vi "Test Zentral Trigger PC nur Mira Sync.vi"() -> ()   [LabVIEW 2009, in "POLARIS BME DG.lvlib"]
uses:
  POLARIS BME DG.lvlib
  LV-BME Interface/ChnlSettings.ctl
  LV-BME Interface/BME_DG_TriggerSettings.ctl
  DG Classes/BME_DG_G05P2/SG05P2 Clock and Trigger Settings.ctl
  LV-BME Interface/ClockSource.ctl
  DG Classes/BME_DG_G05P2/BME_DG_G05P2.lvclass
  DG Classes/BME_DG_G05P2_Chnl/BME_DG_G05P2_Chnl.lvclass
  ChnlParam.ctl
  DG Classes/BME_DG_System/BME_DG_System.lvclass
  DG Classes/BME_DG_Base/BME_DG_Base.lvclass
  DG Classes/BME_DG_Chnl/BME_DG_Chnl.lvclass
panel:
  in  "pathParameterFile":path=path "C:/CS Framework/LVSCC/LV2009/GPL/Projects/cs-framework/CSClass/CSPOLARIS/POLARIS BME DG/tset config  file.xml"
  out "stop error":errorcluster
  in  "Karten Parameter":T1[](array[typedef])=[{"Trigger"={"InputTerminated?"=TRUE, "InternalClockPeriode(µs)"=100000.0, "TriggerLevel"=1.8999000000000001, "PresetValue"=0, "DivideBy"=0, "Clock Source"=1, "Gate Divider"=1, "PositiveGate?"=TRUE, "InternalTrigger?"=TRUE, "InternalArm?"=FALSE, "SWTrigger?"=FALSE, "RisingEdge?"=FALSE, "StopOnPreset?"=FALSE, "ResetWhenDone?"=TRUE, "TriggerEnabled?"=TRUE}, "ClockSource "=1, "V2 Trigger Settings"={"Gate Type"=TRUE, "Synchronize Gate"=FALSE, "Force Trigger (µs)"=0.0, "MS Bus"=1024}, " prescaller crst oscill."=8, "CardName"="Mira Sync"}] {"V2 Trigger Settings"."MS Bus" format="%04x" items=["Local Primary"=1, "Local Secondary"=2, "Local Force"=4, "Resynchronize"=8, "Master Primary"=16, "Master Secondary"=32, "Master Force"=64, "System Clock"=128, "Delay Clock"=256, "Inhibit Local"=512, "Start Local"=1024, "Start Bus"=2048, "Step Back Local"=4096, "Step Back Bus"=8192, "Enable From E"=65536, "Enable From F"=131072, "Enable From Bus"=262144]; "V2 Trigger Settings"."Force Trigger (µs)" min=0.0 format="%.6f"; "ClockSource" items=["Internal Oscillator"=1, "External Trigger"=2, "Trigger & Oscillator"=3, "MasterSlave Bus"=4]; "Trigger"."Gate Divider" min=1 max=1000000; "Trigger"."Clock Source" items=["Internal Oscillator"=1, "External Trigger"=2, "Trigger & Oscillator"=3]; "Trigger"."InternalClockPeriode(µs)" format="%#_11g"}
  in  "Go Signal":u32(ring)=1 items=["Local Primary"=1, "Local Secondary"=2, "Local Force"=4, "Resynchronize"=8, "Master Primary"=16, "Master Secondary"=32, "Master Force"=64, "System Clock"=128, "Delay Clock"=256, "Inhibit Local"=512, "Start Local"=1024, "Start Bus"=2048, "Step Back Local"=4096, "Step Back Bus"=8192, "From E"=65536, "From F"=131072, "From Bus"=262144]
  out "Problem Chnls out":string[](array[string])
  out "DelayFormulas":string[](array[string])=["0.0", "", ""]
  in  "Reset Error":bool
  out "error out":errorcluster
  in  "Update Delay formula":bool=TRUE
  in  "DelayFormula":string="0.0"
  in  "Aknowledge interrupts":bool=TRUE
  in  "stop 3":bool=TRUE
  in  "SetDelay":bool=TRUE
  in  "UpdateChnl":bool=TRUE
  in  "ChnlParameter":T5 {"ChnParam2write"."Delay (µs)" min=0.0 max=100000000.0 format="%.5f"}
  out "CountsRemains":i32=2147483647
  out "TriggerCounters":i32[](array[numeric])=[0, 0, 0, 0, 0, -533591008, 0, 0, 0, 0]
  out "Interrupts":u32[](array[numeric])=[11008, 11008, 10240, 11008, 11008, 11008, 11008, 10240, 10240, 10240] format="%b"
  out "RemainingTriggers":T6(array[cluster])=[[{"Time Stamp"=timestamp(3421635734.171875 s since 1904-01-01), "Numeric"=1}, {"Time Stamp"=timestamp(3421635734.171875 s since 1904-01-01), "Numeric"=1}, {"Time Stamp"=timestamp(3421635734.171875 s since 1904-01-01), "Numeric"=1}, {"Time Stamp"=timestamp(3421635734.171875 s since 1904-01-01), "Numeric"=1}, {"Time Stamp"=timestamp(3421635734.171875 s since 1904-01-01), "Numeric"=1}, {"Time Stamp"=timestamp(3421635734.171875 s since 1904-01-01), "Numeric"=1}, {"Time Stamp"=timestamp(3421635734.171875 s since 1904-01-01), "Numeric"=1}, {"Time Stamp"=timestamp(3421635734.171875 s since 1904-01-01), "Numeric"=1}, {"Time Stamp"=timestamp(3421635734.171875 s since 1904-01-01), "Numeric"=1}, {"Time Stamp"=timestamp(3421635734.171875 s since 1904-01-01), "Numeric"=1}], [{"Time Stamp"=timestamp(3421635734.171875 s since 1904-01-01), "Numeric"=1}, {"Time Stamp"=timestamp(3421635734.171875 s since 1904-01-01), "Numeric"=1}, {"Time Stamp"=timestamp(3421635734.171875 s since 1904-01-01), "Numeric"=1}, {"Time Stamp"=timestamp(3421635734.171875 s since 1904-01-01), "Numeric"=1}, {"Time Stamp"=timestamp(3421635734.171875 s since 1904-01-01), "Numeric"=1}, {"Time Stamp"=timestamp(3421635734.171875 s since 1904-01-01), "Numeric"=1}, {"Time Stamp"=timestamp(3421635734.171875 s since 1904-01-01), "Numeric"=1}, {"Time Stamp"=timestamp(3421635734.171875 s since 1904-01-01), "Numeric"=1}, {"Time Stamp"=timestamp(3421635734.171875 s since 1904-01-01), "Numeric"=1}, {"Time Stamp"=timestamp(3421635734.171875 s since 1904-01-01), "Numeric"=1}], [{"Time Stamp"=timestamp(3421635734.171875 s since 1904-01-01), "Numeric"=1}, {"Time Stamp"=timestamp(3421635734.171875 s since 1904-01-01), "Numeric"=1}, {"Time Stamp"=timestamp(3421635734.171875 s since 1904-01-01), "Numeric"=1}, {"Time Stamp"=timestamp(3421635734.171875 s since 1904-01-01), "Numeric"=1}, {"Time Stamp"=timestamp(3421635734.171875 s since 1904-01-01), "Numeric"=1}, {"Time Stamp"=timestamp(3421635734.171875 s since 1904-01-01), "Numeric"=1}, {"Time Stamp"=timestamp(3421635734.171875 s since 1904-01-01), "Numeric"=1}, {"Time Stamp"=timestamp(3421635734.171875 s since 1904-01-01), "Numeric"=1}, {"Time Stamp"=timestamp(3421635734.171875 s since 1904-01-01), "Numeric"=1}, {"Time Stamp"=timestamp(3421635734.171875 s since 1904-01-01), "Numeric"=1}]] {"Time Stamp" format="%<%I:%M:%S%3u %p>T"}
  in  "stop 2":bool=TRUE
  in  "ReadStatus":bool=TRUE
  in  "Activate":bool=TRUE
  in  "ResetModuloCounters":bool=TRUE
  in  "TriggerModulo":u32=4
  out "Modulo Settings":u32[](array[numeric])=[1, 1, 1]
  out "Chnls":T4[](array[typedef])=[{" Delay (µs)"=0.0, "On? (false)"=TRUE, "PositiveVoltage?"=TRUE, "50OhmTerminated? "=TRUE, "25OhmOutput?"=FALSE}, {" Delay (µs)"=0.0, "On? (false)"=TRUE, "PositiveVoltage?"=TRUE, "50OhmTerminated? "=TRUE, "25OhmOutput?"=FALSE}, {" Delay (µs)"=0.0, "On? (false)"=TRUE, "PositiveVoltage?"=TRUE, "50OhmTerminated? "=TRUE, "25OhmOutput?"=FALSE}] {"Delay (µs)" min=0.0 max=100000000.0 format="%.5f"}
  in  "Trigger Base":T2={"InputTerminated?"=TRUE, "InternalClockPeriode(µs)"=100000.0, "TriggerLevel"=-0.1001, "PresetValue"=0, "DivideBy"=4, "Clock Source"=1, "Gate Divider"=1, "PositiveGate?"=TRUE, "InternalTrigger?"=TRUE, "InternalArm?"=FALSE, "SWTrigger?"=FALSE, "RisingEdge?"=FALSE, "StopOnPreset?"=FALSE, "ResetWhenDone?"=TRUE, "TriggerEnabled?"=TRUE} {"Gate Divider" min=1 max=1000000; "Clock Source" items=["Internal Oscillator"=1, "External Trigger"=2, "Trigger & Oscillator"=3]; "InternalClockPeriode(µs)" format="%#_11g"}
  in  "Selected Chnl":u16(ring) items=["18 MHz", "A", "B"]
  in  "Selected Card":u16(ring) items=["Mira Sync"]
  in  "STOP":bool=TRUE
  in  "ChnParam2write":T4={" Delay (µs)"=0.0, "On? (false)"=TRUE, "PositiveVoltage?"=TRUE, "50OhmTerminated? "=TRUE, "25OhmOutput?"=FALSE} {"Delay (µs)" min=0.0 max=100000000.0 format="%.5f"}
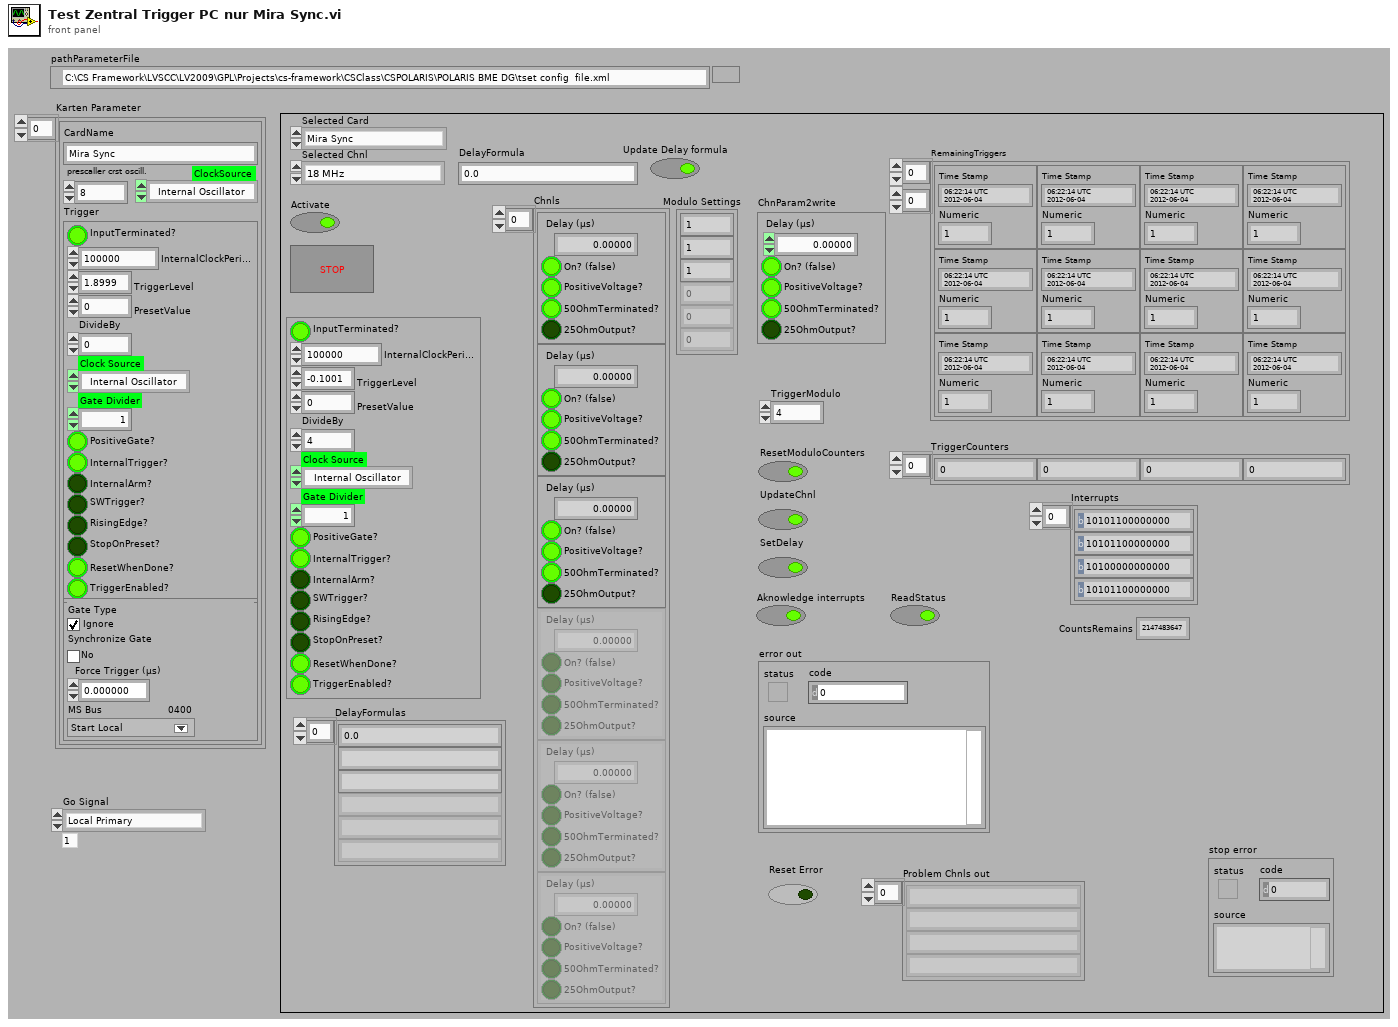
[diagram p1: front panel]
types:
  T1 = typedef "SG05P2 Clock and Trigger Settings.ctl" = cluster{"Trigger":T2, "ClockSource ":T3, "V2 Trigger Settings":cluster{"Gate Type":bool, "Synchronize Gate":bool, "Force Trigger (µs)":dbl, "MS Bus":u32}, " prescaller crst oscill.":u32, "CardName":string}
  T2 = typedef "POLARIS BME DG.lvlib/BME_DG_TriggerSettings.ctl" = cluster{"InputTerminated?":bool, "InternalClockPeriode(µs)":dbl, "TriggerLevel":dbl, "PresetValue":i32, "DivideBy":i32, "Clock Source":u32, "Gate Divider":i32, "PositiveGate?":bool, "InternalTrigger?":bool, "InternalArm?":bool, "SWTrigger?":bool, "RisingEdge?":bool, "StopOnPreset?":bool, "ResetWhenDone?":bool, "TriggerEnabled?":bool}
  T3 = typedef "POLARIS BME DG.lvlib/ClockSource.ctl" = i32
  T4 = typedef "POLARIS BME DG.lvlib/ChnlSettings.ctl" = cluster{" Delay (µs)":dbl, "On? (false)":bool, "PositiveVoltage?":bool, "50OhmTerminated? ":bool, "25OhmOutput?":bool}
  T5 = cluster{"ChnlName":string, "ChnParam2write":T4, "TriggerModulo":u32}
  T6 = cluster{"Time Stamp":timestamp, "Numeric":i32}[][]
  T7 = typedef "ChnlParam.ctl" = cluster{"ChnlName":string, "DelayFormula":string, "OutputModulo":i32}
  T8 = cluster{"Gate Type":bool, "Synchronize Gate":bool, "Force Trigger (µs)":dbl, "MS Bus":u32}
  T9 = enum8{"Enabled", "Disabled", "Disabled and Grayed Out"}
  T10 = cluster{"ChnlName":string, "ChnParam2write":T4, "TriggerModulo":u32}[]
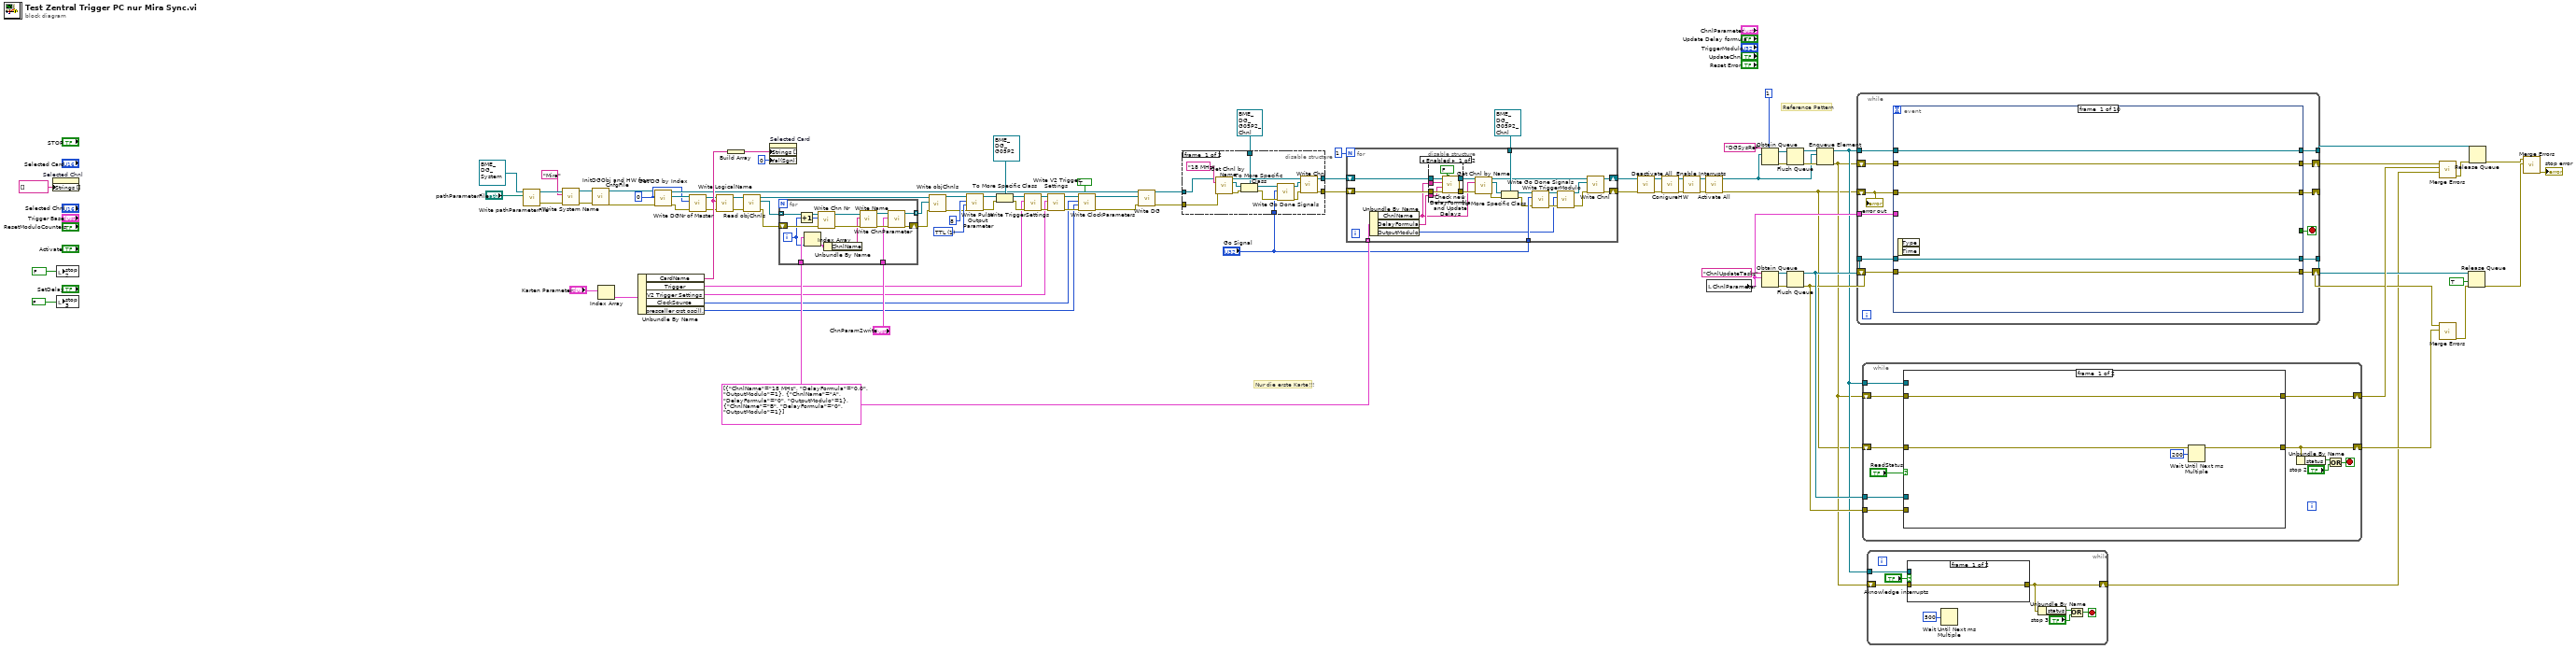
[diagram p0: block diagram]
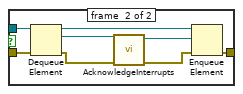
[diagram p4: hidden frame]
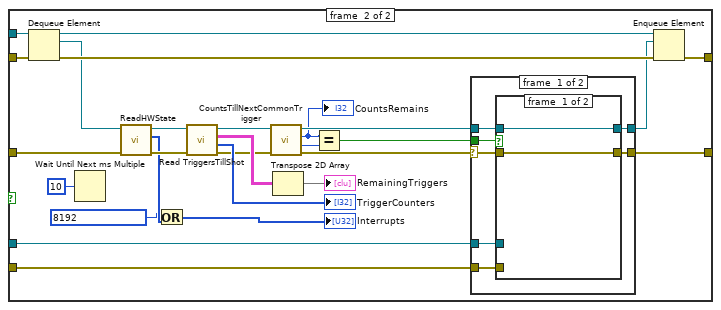
[diagram p5: hidden frame]
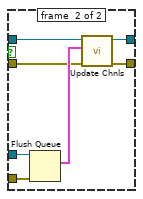
[diagram p6: hidden frame]
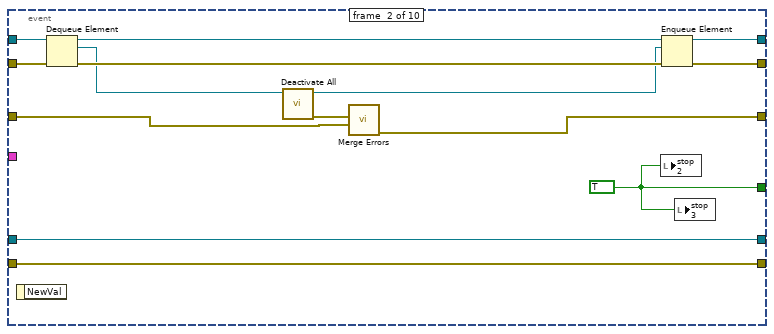
[diagram p8: hidden frame]
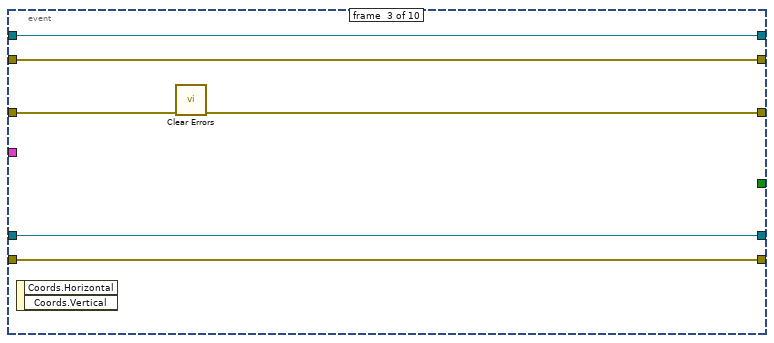
[diagram p9: hidden frame]
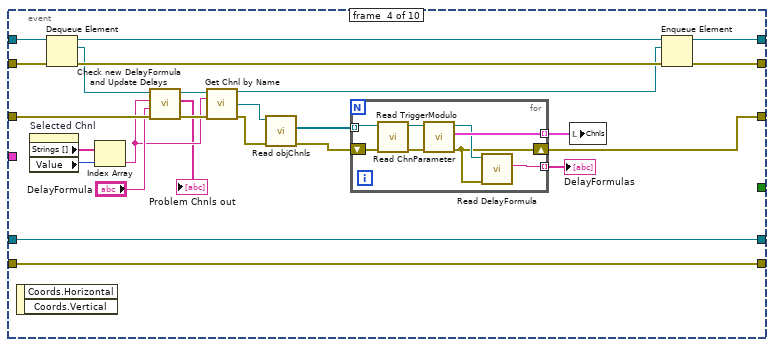
[diagram p10: hidden frame]
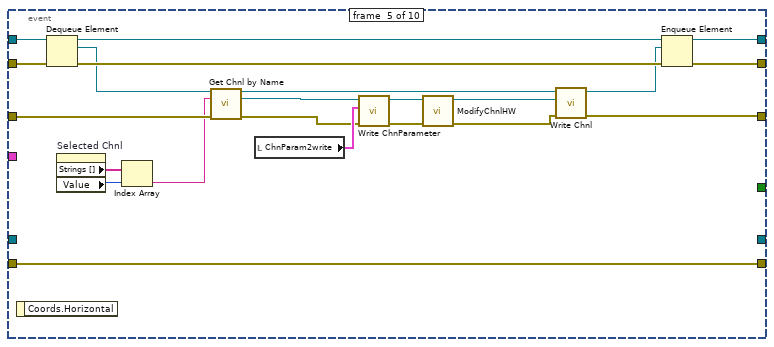
[diagram p11: hidden frame]
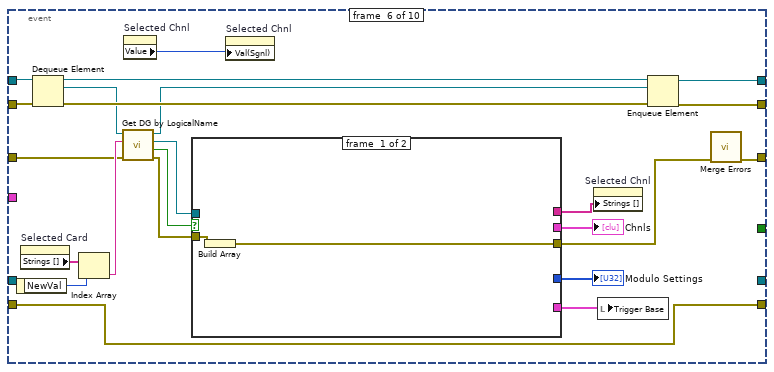
[diagram p12: hidden frame]
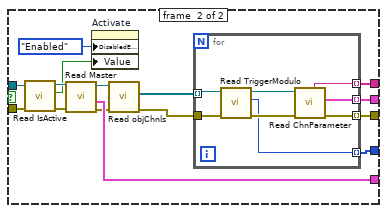
[diagram p13: hidden frame]
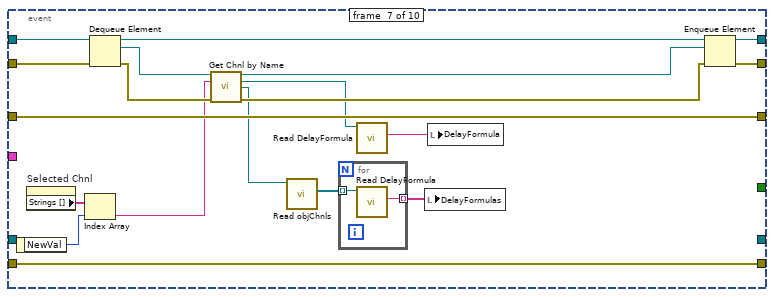
[diagram p14: hidden frame]
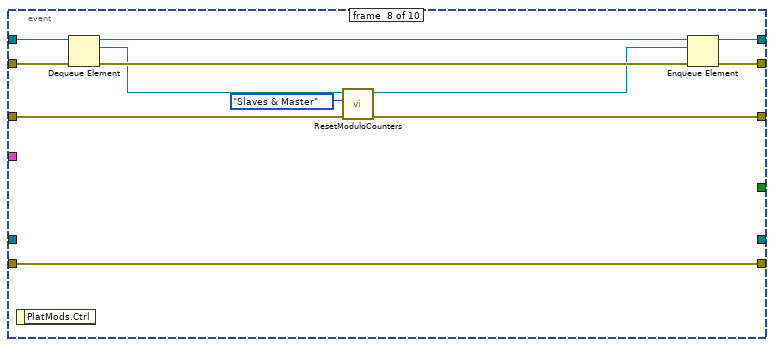
[diagram p15: hidden frame]
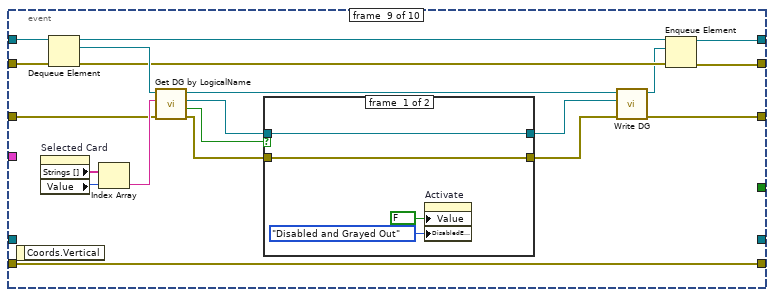
[diagram p16: hidden frame]
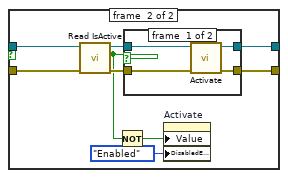
[diagram p17: hidden frame]
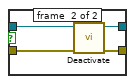
[diagram p18: hidden frame]
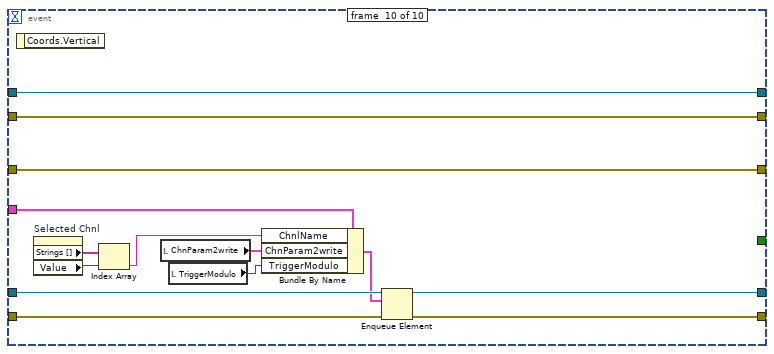
[diagram p19: hidden frame]
diagram:
  w31 = u32 1 items=["TTL"=1, "NIM"=2, "ECL"=3] ("Pulse Output Level")
  w46 = T7[] [{"ChnlName"="18 MHz", "DelayFormula"="0.0", "OutputModulo"=1}, {"ChnlName"="A", "DelayFormula"="0", "OutputModulo"=1}, {"ChnlName"="B", "DelayFormula"="0", "OutputModulo"=1}] ("ChnlParam 2")
  w10 = 0
  # "Nur die erste Karte!!!"
  # "Reference Pattern"
  n1 = property on="Selected Chnl" class="Ring (strict)"("Strings []"=string[] []) -> ()  [unwired: 2 in, 2 out]
  n2 = local write "stop 2"(FALSE ("stop 2")) -> ()
  n3 = local write "stop 3"(FALSE ("stop 3")) -> ()
  n4 = call-dynamic "Write pathParameterFile.vi"("pathParameterFile"="pathParameterFile", "BME_DG_System in"=refnum<class "BME_DG_System.lvclass"> refnum) -> ("error out"=w6:errorcluster, "BME_DG_System out"=w7:refnum<class "BME_DG_System.lvclass">)  [unwired: 8 in]
  n5 = call "Write System Name.vi"("error in (no error)"=w6, "log Name"="Mira", "BME_DG_System in"=w7) -> ("error out"=w3:errorcluster, "BME_DG_System out"=w4:refnum<class "BME_DG_System.lvclass">)  [unwired: 7 in]
  n6 = call "InitDGObj and HW from CnfgFile.vi"("error out"=w3, "BME_DG_System in"=w4) -> ("error IO"=w1:errorcluster, "BME_DG_System Out"=w2:refnum<class "BME_DG_System.lvclass">)  [unwired: 4 in]
  n7 = Index Array(array="Karten Parameter") -> (element=w14:T1)  [unwired: 1 in]
  n8 = Unbundle By Name(w14) -> ("CardName"=w72:string, "Trigger"=w18:T2, "V2 Trigger Settings"=w17:T8, "ClockSource"=w15:T3, "prescaller crst oscill."=w16:u32)
  n9 = call "Get DG by Index.vi"("error in (no error)"=w1, "index"=w10, "BME_DG_System in"=w2) -> ("error out"=w34:errorcluster, "BME_DG_Base.lvclass"=w37:refnum<class "BME_DG_Base.lvclass">, "BME_DG_System out"=w45:refnum<class "BME_DG_System.lvclass">)  [unwired: 6 in]
  n10 = call-dynamic "Write DGNr of Master.vi"("error in (no error)"=w34, "DGNr of Master"=w10, "BME_DG_Base in"=w37) -> ("error out"=w35:errorcluster, "BME_DG_Base out"=w36:refnum<class "BME_DG_Base.lvclass">)  [unwired: 7 in]
  n11 = call "Write LogicalName.vi"("error in (no error)"=w35, "LogicalName"=w72, "BME_DG_Base in"=w36) -> ("error out"=w38:errorcluster, "BME_DG_Base out"=w39:refnum<class "BME_DG_Base.lvclass">)  [unwired: 7 in]
  n12 = Build Array(w72) -> (w13:string[])
  n13 = call-dynamic "Read objChnls.vi"("error in (no error)"=w38, "BME_DG_Base in"=w39) -> ("error out"=w43:errorcluster, "objChnls"=w44:refnum<class "BME_DG_Chnl.lvclass">[], "BME_DG_Base out"=w41:refnum<class "BME_DG_Base.lvclass">)  [unwired: 6 in, 1 out]
  n14 = property on="Selected Card" class="Ring (strict)"("Strings []"=w13, "Val(Sgnl)"=u16 0 ("Value (Signaling)")) -> ()  [unwired: 2 in, 2 out]
  n15 = for {
    tunnel: w44 -> [w108] mode=indexing
    shift-right: [w100] -> w40
    shift-left: w43 -> [w106]
    tunnel: "ChnParam2write" -> [w109]
    tunnel: [w101] -> w42 mode=indexing
    tunnel: w46 -> [w103]
    i -> [w99]
    n16 = Increment(x=w99) -> (x+1=w104:i32)
    n17 = Index Array(array=w103, index=w99) -> (element=w102:T7)
    n18 = call-dynamic "Write Chn Nr.vi"("error in (no error)"=w106, "Chn Nr"=w104, "BME_DG_Chnl in"=w108) -> ("error out"=w105:errorcluster, "BME_DG_Chnl out"=w107:refnum<class "BME_DG_Chnl.lvclass">)  [unwired: 7 in]
    n19 = Unbundle By Name(w102) -> ("ChnlName"=w98:string)
    n20 = call-dynamic "Write Name.vi"("error in (no error)"=w105, "Name"=w98, "BME_DG_Chnl in"=w107) -> ("error out"=w110:errorcluster, "BME_DG_Chnl out"=w111:refnum<class "BME_DG_Chnl.lvclass">)  [unwired: 7 in]
    n21 = call-dynamic "Write ChnParameter.vi"("error in (no error)"=w110, "ChnParemater"=w109, "BME_DG_Chnl in"=w111) -> ("error out"=w100:errorcluster, "BME_DG_Chnl out"=w101:refnum<class "BME_DG_Chnl.lvclass">)  [unwired: 7 in]
  }
  n22 = call-dynamic "Write objChnls.vi"("error in (no error)"=w40, "objChnls"=w42, "BME_DG_Base in"=w41) -> ("error out"=w30:errorcluster, "BME_DG_Base out"=w33:refnum<class "BME_DG_Base.lvclass">)  [unwired: 7 in]
  n23 = call-dynamic "Write Pulse Output Parameter.vi"("error in (no error)"=w30, "Pulse Output Level"=w31, "Pulse Width"=u32 8, "BME_DG_Base in"=w33) -> ("error out"=w21:errorcluster, "BME_DG_Base out"=w23:refnum<class "BME_DG_Base.lvclass">)  [unwired: 6 in]
  n24 = To More Specific Class(target class=refnum<class "BME_DG_G05P2.lvclass"> refnum ("BME_DG_G05P2.lvclass"), reference=w23, error in=w21) -> (specific class reference=w24:refnum<class "BME_DG_G05P2.lvclass">, error out=w25:errorcluster)
  n25 = call-dynamic "Write TriggerSettings.vi"("error in (no error)"=w25, "Trigger Settings"=w18, "BME_DG_Base in"=w24) -> ("error out"=w28:errorcluster, "BME_DG_Base out"=w26:refnum<class "BME_DG_G05P2.lvclass">)  [unwired: 7 in]
  n26 = call-dynamic "Write V2 Trigger Settings.vi"("error in (no error)"=w28, "V2 Trigger Settings"=w17, "BME_DG_G05 in"=w26) -> ("error out"=w29:errorcluster, "BME_DG_G05 out"=w27:refnum<class "BME_DG_G05P2.lvclass">)  [unwired: 7 in]
  n27 = call-dynamic "Write ClockParameters.vi"("ClockEnable"=TRUE, "error in (no error)"=w29, "PrescalerCrystalOscilator"=w16, "ClockSource"=w15, "BME_DG_Base in"=w27) -> ("error out"=w20:errorcluster, "BME_DG_Base out"=w22:refnum<class "BME_DG_G05P2.lvclass">)  [unwired: 5 in]
  n28 = call "Write DG.vi"("error in (no error)"=w20, "BME_DG_Base"=w22, "BME_DG_System in"=w45) -> ("error out"=w53:errorcluster, "BME_DG_System out"=w54:refnum<class "BME_DG_System.lvclass">)  [unwired: 7 in]
  n29 = disable-structure shown="Enabled" {
    disable-tunnel: refnum<class "BME_DG_G05P2_Chnl.lvclass"> refnum ("BME_DG_G05P2_Chnl.lvclass") -> [w121 _]
    disable-tunnel: w54 -> [w116 w127]
    disable-tunnel: w53 -> [w115 w126]
    disable-tunnel: [w114 w127] -> w51
    disable-tunnel: [w113 w126] -> w50
    disable-tunnel: "Go Signal" -> [w112 _]
    frame #0 {
      n30 = call "Get Chnl by Name.vi"("BME_DG_System in"=w116, "Chnl Name"="18 MHz", "error in (no error)"=w115) -> ("BME_DG_System out"=w124:refnum<class "BME_DG_System.lvclass">, "BME_DG_Chnl"=w123:refnum<class "BME_DG_Chnl.lvclass">, "error out"=w120:errorcluster)  [unwired: 7 in, 3 out]
      n31 = To More Specific Class(target class=w121, reference=w123, error in=w120) -> (specific class reference=w122:refnum<class "BME_DG_G05P2_Chnl.lvclass">, error out=w119:errorcluster)
      n32 = call-dynamic "Write Go Done Signals.vi"("error in (no error)"=w119, "Go Signal"=w112, "BME_DG_G05P2_Chnl in"=w122) -> ("error out"=w118:errorcluster, "BME_DG_G05P2_Chnl out"=w117:refnum<class "BME_DG_G05P2_Chnl.lvclass">)  [unwired: 7 in]
      n33 = call "Write Chnl.vi"("error in (no error)"=w118, "BME_DG_Chnl.lvclass"=w117, "BME_DG_System in"=w124) -> ("error out"=w113:errorcluster, "BME_DG_System out"=w114:refnum<class "BME_DG_System.lvclass">)  [unwired: 7 in]
    }
    frame #1 {
    }
  }
  n34 = for {
    N: 1 -> [_]
    shift-right: [w132] -> w58
    shift-left: w51 -> [w148]
    shift-right: [w131] -> w57
    shift-left: w50 -> [w147]
    tunnel: w46 -> [w146] mode=indexing
    tunnel: refnum<class "BME_DG_G05P2_Chnl.lvclass"> refnum ("BME_DG_G05P2_Chnl.lvclass") -> [w140]
    tunnel: "Go Signal" -> [w138]
    n35 = Unbundle By Name(w146) -> ("ChnlName"=w142:string, "DelayFormula"=w145:string, "OutputModulo"=w133:i32)
    n36 = disable-structure shown="Enabled" {
      disable-tunnel: w148 -> [w155 w157]
      disable-tunnel: w147 -> [w154 w156]
      disable-tunnel: w145 -> [w152 _]
      disable-tunnel: [w151 w157] -> w144
      disable-tunnel: [w150 w156] -> w143
      disable-tunnel: w142 -> [w149 _]
      frame #0 {
        n37 = call "Check new DelayFormula and Update Delays.vi"("Update HW"=FALSE, "error in (no error)"=w154, "Delay Formula"=w152, "ChnlName"=w149, "BME_DG_System in"=w155) -> ("error out"=w150:errorcluster, "BME_DG_System out"=w151:refnum<class "BME_DG_System.lvclass">)  [unwired: 4 in, 1 out]
      }
      frame #1 {
      }
    }
    n38 = call "Get Chnl by Name.vi"("BME_DG_System in"=w144, "Chnl Name"=w142, "error in (no error)"=w143) -> ("BME_DG_System out"=w130:refnum<class "BME_DG_System.lvclass">, "BME_DG_Chnl"=w139:refnum<class "BME_DG_Chnl.lvclass">, "error out"=w137:errorcluster)  [unwired: 7 in, 3 out]
    n39 = To More Specific Class(target class=w140, reference=w139, error in=w137) -> (specific class reference=w141:refnum<class "BME_DG_G05P2_Chnl.lvclass">, error out=w136:errorcluster)
    n40 = call-dynamic "Write Go Done Signals.vi"("error in (no error)"=w136, "Go Signal"=w138, "BME_DG_G05P2_Chnl in"=w141) -> ("error out"=w134:errorcluster, "BME_DG_G05P2_Chnl out"=w135:refnum<class "BME_DG_G05P2_Chnl.lvclass">)  [unwired: 7 in]
    n41 = call-dynamic "Write TriggerModulo.vi"("error in (no error)"=w134, "TriggerModulo"=w133, "BME_DG_G05_Chnl in"=w135) -> ("error out"=w129:errorcluster, "BME_DG_G05_Chnl out"=w128:refnum<class "BME_DG_G05P2_Chnl.lvclass">)  [unwired: 7 in]
    n42 = call "Write Chnl.vi"("error in (no error)"=w129, "BME_DG_Chnl.lvclass"=w128, "BME_DG_System in"=w130) -> ("error out"=w131:errorcluster, "BME_DG_System out"=w132:refnum<class "BME_DG_System.lvclass">)  [unwired: 7 in]
  }
  n43 = call "Deactivate All.vi"("error in (no error)"=w57, "BME_DG_System in"=w58) -> ("error out"=w70:errorcluster, "BME_DG_System out"=w71:refnum<class "BME_DG_System.lvclass">)  [unwired: 8 in]
  n44 = call "ConigureHW.vi"("error in (no error)"=w70, "BME_DG_System in"=w71) -> ("error out"=w68:errorcluster, "BME_DG_System out"=w69:refnum<class "BME_DG_System.lvclass">)  [unwired: 8 in]
  n45 = call "Enable Interrupts.vi"("error in (no error)"=w68, "BME_DG_System in"=w69) -> ("error out"=w62:errorcluster, "BME_DG_System out"=w63:refnum<class "BME_DG_System.lvclass">)  [unwired: 8 in]
  n46 = call "Activate All.vi"("error in (no error)"=w62, "BME_DG_System in"=w63) -> ("error out"=w60:errorcluster, "BME_DG_System out"=w61:refnum<class "BME_DG_System.lvclass">)  [unwired: 8 in]
  n47 = local read "ChnlParameter"() -> (w80:T5)
  n48 = Obtain Queue(max queue size (-1, unlimited)=1, name (unnamed)="DGSysRef", element data type=w61) -> (queue out=w88:refnum<queue>, error out=w86:errorcluster)  [unwired: 2 in, 1 out]
  n49 = Obtain Queue(name (unnamed)="ChnlUpdateTasks", element data type=w80) -> (queue out=w81:refnum<queue>, error out=w82:errorcluster)  [unwired: 3 in, 1 out]
  n50 = Flush Queue(queue=w88, error in (no error)=w86) -> (queue out=w87:refnum<queue>, error out=w85:errorcluster)  [unwired: 1 out]
  n51 = Flush Queue(queue=w81, error in (no error)=w82) -> (queue out=w77:refnum<queue>, error out=w76:errorcluster)  [unwired: 1 out]
  n52 = Enqueue Element(queue=w87, element=w61, error in (no error)=w85) -> (queue out=w67:refnum<queue>, error out=w66:errorcluster)  [unwired: 1 in, 1 out]
  n53 = while {
    shift-right: [w165] -> _
    shift-left: w60 -> [w167]
    shift-right: [w163] -> w91
    shift-left: w66 -> [w164]
    tunnel: w67 -> [w168]
    tunnel: [w166] -> w93
    tunnel: w77 -> [w162]
    tunnel: w80 -> [w161]
    tunnel: [w159] -> w79
    shift-right: [w158] -> w75
    shift-left: w76 -> [w160]
    stop <- w169 stop-if-true
    n54 = event shown="[5] \"Selected Card\": Value Change" {
      selector: _ -> [_ _ _ _ _ _ _ _ _ _]
      dyn-events: _ -> [_ _ _ _ _ _ _ _ _ _]
      timeout: _ -> [_ _ _ _ _ _ _ _ _ _]
      tunnel: [_ w177 _ _ _ _ _ _ _ _] -> w169
      tunnel: w168 -> [w174 w186 w193 w218 w248 w260 w311 w330 w339 w385]
      tunnel: w167 -> [w173 w175 w194 w210 w239 w269 w316 w320 w347 w384]
      tunnel: [w174 w182 w193 w214 w244 w258 w309 w325 w333 w385] -> w166
      tunnel: [w173 w176 w189 w198 w228 w253 w316 w321 w340 w384] -> w165
      tunnel: w164 -> [w172 w185 w192 w217 w247 w259 w310 w328 w338 w381]
      tunnel: [w172 w183 w192 w215 w245 w257 w308 w326 w332 w381] -> w163
      tunnel: w162 -> [w171 w179 w191 w213 _ _ _ _ _ w376]
      tunnel: w161 -> [_ _ _ _ _ _ _ _ _ w380]
      tunnel: w160 -> [w170 w178 w190 w212 w243 w251 w315 w324 w331 w374]
      tunnel: [w171 w179 w191 w213 _ _ _ _ _ w373] -> w159
      tunnel: [w170 w178 w190 w212 w243 w251 w315 w324 w331 w372] -> w158
      event #0 {
        n55 = event-data() -> ()  [unwired: 1 in, 2 out]
      }
      event #1 {
        w177 = TRUE
        n56 = event-data() -> ()  [unwired: 1 in, 1 out]
        n57 = Dequeue Element(queue=w186, error in (no error)=w185) -> (queue out=w187:refnum<queue>, element=w180:refnum<class "BME_DG_System.lvclass">, error out=w184:errorcluster)  [unwired: 1 in, 1 out]
        n58 = call "Deactivate All.vi"("BME_DG_System in"=w180) -> ("error out"=w188:errorcluster, "BME_DG_System out"=w181:refnum<class "BME_DG_System.lvclass">)  [unwired: 9 in]
        n59 = call <vilib>:"Merge Errors.vi"("error in 3 (no error)"=w175, "error in 2 (no error)"=w188) -> ("error out"=w176:errorcluster)  [unwired: 5 in]
        n60 = local write "stop 2"(w177) -> ()
        n61 = Enqueue Element(queue=w187, element=w181, error in (no error)=w184) -> (queue out=w182:refnum<queue>, error out=w183:errorcluster)  [unwired: 1 in, 1 out]
        n62 = local write "stop 3"(w177) -> ()
      }
      event #2 {
        n63 = event-data() -> ()  [unwired: 1 in, 2 out]
        n64 = call <vilib>:"Clear Errors.vi"("error in (no error)"=w194) -> ("error out"=w189:errorcluster)  [unwired: 6 in]
      }
      event #3 {
        n65 = event-data() -> ()  [unwired: 1 in, 2 out]
        n66 = property on="Selected Chnl" class="Ring (strict)"() -> ("Strings []"=w208:string[], "Value"=w209:u16)  [unwired: 2 in, 2 out]
        n67 = Dequeue Element(queue=w218, error in (no error)=w217) -> (queue out=w219:refnum<queue>, element=w211:refnum<class "BME_DG_System.lvclass">, error out=w216:errorcluster)  [unwired: 1 in, 1 out]
        n68 = Index Array(array=w208, index=w209) -> (element=w197:string)
        n69 = call "Check new DelayFormula and Update Delays.vi"("error in (no error)"=w210, "Delay Formula"="DelayFormula", "ChnlName"=w197, "BME_DG_System in"=w211) -> ("error out"=w200:errorcluster, "Problem Chnls out"=→"Problem Chnls out":string[], "BME_DG_System out"=w202:refnum<class "BME_DG_System.lvclass">)  [unwired: 5 in]
        n70 = call "Get Chnl by Name.vi"("BME_DG_System in"=w202, "Chnl Name"=w197, "error in (no error)"=w200) -> ("BME_DG_System out"=w201:refnum<class "BME_DG_System.lvclass">, "Owner DG"=w203:refnum<class "BME_DG_Base.lvclass">, "error out"=w199:errorcluster)  [unwired: 7 in, 3 out]
        n71 = call-dynamic "Read objChnls.vi"("error in (no error)"=w199, "BME_DG_Base in"=w203) -> ("error out"=w204:errorcluster, "objChnls"=w206:refnum<class "BME_DG_Chnl.lvclass">[])  [unwired: 6 in, 2 out]
        n72 = for {
          tunnel: w206 -> [w226] mode=indexing
          tunnel: [w227] -> w205 mode=indexing
          shift-right: [w221] -> w198
          shift-left: w204 -> [w224]
          tunnel: [w220] -> w196 mode=indexing
          n73 = call-dynamic "Read TriggerModulo.vi"("error in (no error)"=w224, "BME_DG_Chnl in"=w226) -> ("error out"=w223:errorcluster, "BME_DG_Chnl out"=w225:refnum<class "BME_DG_Chnl.lvclass">)  [unwired: 7 in, 1 out]
          n74 = call-dynamic "Read ChnParameter.vi"("error in (no error)"=w223, "BME_DG_Chnl in"=w225) -> ("error out"=w221:errorcluster, "ChnParemater"=w227:T4, "BME_DG_Chnl out"=w222:refnum<class "BME_DG_Chnl.lvclass">)  [unwired: 4 in, 3 out]
          n75 = call-dynamic "Read DelayFormula.vi"("error in (no error)"=w221, "BME_DG_Chnl in"=w222) -> ("DelayFormula"=w220:string)  [unwired: 7 in, 2 out]
        }
        "DelayFormulas" <- w196
        n76 = local write "Chnls"(w205) -> ()
        n77 = Enqueue Element(queue=w219, element=w201, error in (no error)=w216) -> (queue out=w214:refnum<queue>, error out=w215:errorcluster)  [unwired: 1 in, 1 out]
      }
      event #4 {
        n78 = event-data() -> ()  [unwired: 1 in, 1 out]
        n79 = Dequeue Element(queue=w248, error in (no error)=w247) -> (queue out=w249:refnum<queue>, element=w240:refnum<class "BME_DG_System.lvclass">, error out=w246:errorcluster)  [unwired: 1 in, 1 out]
        n80 = property on="Selected Chnl" class="Ring (strict)"() -> ("Strings []"=w241:string[], "Value"=w242:u16)  [unwired: 2 in, 2 out]
        n81 = Index Array(array=w241, index=w242) -> (element=w238:string)
        n82 = call "Get Chnl by Name.vi"("BME_DG_System in"=w240, "Chnl Name"=w238, "error in (no error)"=w239) -> ("BME_DG_System out"=w234:refnum<class "BME_DG_System.lvclass">, "BME_DG_Chnl"=w237:refnum<class "BME_DG_Chnl.lvclass">, "error out"=w235:errorcluster)  [unwired: 7 in, 3 out]
        n83 = local read "ChnParam2write"() -> (w236:T4)
        n84 = call-dynamic "Write ChnParameter.vi"("error in (no error)"=w235, "ChnParemater"=w236, "BME_DG_Chnl in"=w237) -> ("error out"=w231:errorcluster, "BME_DG_Chnl out"=w232:refnum<class "BME_DG_Chnl.lvclass">)  [unwired: 7 in]
        n85 = call-dynamic "ModifyChnlHW.vi"("error in (no error)"=w231, "BME_DG_Chnl in"=w232) -> ("error out"=w229:errorcluster, "BME_DG_Chnl out"=w230:refnum<class "BME_DG_Chnl.lvclass">)  [unwired: 8 in]
        n86 = call "Write Chnl.vi"("error in (no error)"=w229, "BME_DG_Chnl.lvclass"=w230, "BME_DG_System in"=w234) -> ("error out"=w228:errorcluster, "BME_DG_System out"=w233:refnum<class "BME_DG_System.lvclass">)  [unwired: 7 in]
        n87 = Enqueue Element(queue=w249, element=w233, error in (no error)=w246) -> (queue out=w244:refnum<queue>, error out=w245:errorcluster)  [unwired: 1 in, 1 out]
      }
      event #5 {
        n88 = event-data() -> ("NewVal"=w271:u16)  [unwired: 1 in]
        n89 = property on="Selected Card" class="Ring (strict)"() -> ("Strings []"=w272:string[])  [unwired: 2 in, 2 out]
        n90 = Dequeue Element(queue=w260, error in (no error)=w259) -> (queue out=w261:refnum<queue>, element=w256:refnum<class "BME_DG_System.lvclass">, error out=w262:errorcluster)  [unwired: 1 in, 1 out]
        n91 = Index Array(array=w272, index=w271) -> (element=w270:string)
        n92 = call "Get DG by LogicalName.vi"("error in (no error)"=w269, "LogicalName"=w270, "BME_DG_System in"=w256) -> ("error out"=w254:errorcluster, "found?"=w268:bool, "BME_DG_Base.lvclass"=w267:refnum<class "BME_DG_Base.lvclass">, "BME_DG_System out"=w255:refnum<class "BME_DG_System.lvclass">)  [unwired: 5 in]
        n93 = property on="Selected Chnl" class="Ring (strict)"() -> ("Value"=w250:u16)  [unwired: 2 in, 2 out]
        n94 = case shown="True" w268 {
          tunnel: w267 -> [_ w282]
          tunnel: [_ w289] -> w266
          tunnel: [_ w288] -> w264
          tunnel: [_ w287] -> w265
          tunnel: [_ w283] -> w263
          tunnel: w254 -> [w274 w279]
          tunnel: [w273 w277] -> w252
          frame #0 {
            n95 = Build Array(w274) -> (w273:errorcluster[])
          }
          frame #1 {
            n96 = call-dynamic "Read IsActive.vi"("error in (no error)"=w279, "BME_DG_Base in"=w282) -> ("error out"=w280:errorcluster, "Active?"=w275:bool, "BME_DG_Base out"=w281:refnum<class "BME_DG_Base.lvclass">)  [unwired: 7 in]
            n97 = call-dynamic "Read Master.vi"("error in (no error)"=w280, "BME_DG_Base in"=w281) -> ("error out"=w284:errorcluster, "TriggerSettings"=w287:T2, "BME_DG_Base out"=w285:refnum<class "BME_DG_Base.lvclass">)  [unwired: 6 in, 1 out]
            n98 = property on="Activate" class="Bool (strict)"("DisabledEnum"=T9."Enabled" ("Disabled"), "Value"=w275) -> ()  [unwired: 2 in, 2 out]
            n99 = call-dynamic "Read objChnls.vi"("error in (no error)"=w284, "BME_DG_Base in"=w285) -> ("error out"=w278:errorcluster, "objChnls"=w286:refnum<class "BME_DG_Chnl.lvclass">[])  [unwired: 6 in, 2 out]
            n100 = for {
              tunnel: w286 -> [w295] mode=indexing
              tunnel: [w297] -> w289 mode=indexing
              tunnel: [w296] -> w288 mode=indexing
              tunnel: [w290] -> w283 mode=indexing
              tunnel: w278 -> [w293]
              tunnel: [w291] -> w277 mode=indexing
              n101 = call-dynamic "Read TriggerModulo.vi"("error in (no error)"=w293, "BME_DG_Chnl in"=w295) -> ("error out"=w292:errorcluster, "TriggerModulo"=w290:i32, "BME_DG_Chnl out"=w294:refnum<class "BME_DG_Chnl.lvclass">)  [unwired: 7 in]
              n102 = call-dynamic "Read ChnParameter.vi"("error in (no error)"=w292, "BME_DG_Chnl in"=w294) -> ("error out"=w291:errorcluster, "ChnParemater"=w296:T4, "Name"=w297:string)  [unwired: 4 in, 3 out]
            }
          }
        }
        "Chnls" <- w264
        "Modulo Settings" <- w263
        n103 = property on="Selected Chnl" class="Ring (strict)"("Val(Sgnl)"=w250) -> ()  [unwired: 2 in, 2 out]
        n104 = property on="Selected Chnl" class="Ring (strict)"("Strings []"=w266) -> ()  [unwired: 2 in, 2 out]
        n105 = local write "Trigger Base"(w265) -> ()
        n106 = Enqueue Element(queue=w261, element=w255, error in (no error)=w262) -> (queue out=w258:refnum<queue>, error out=w257:errorcluster)  [unwired: 1 in, 1 out]
        n107 = call <vilib>:"Merge Errors.vi"("error array in"=w252) -> ("error out"=w253:errorcluster)  [unwired: 6 in]
      }
      event #6 {
        n108 = event-data() -> ("NewVal"=w313:u16)  [unwired: 1 in]
        n109 = property on="Selected Chnl" class="Ring (strict)"() -> ("Strings []"=w314:string[])  [unwired: 2 in, 2 out]
        n110 = Index Array(array=w314, index=w313) -> (element=w303:string)
        n111 = Dequeue Element(queue=w311, error in (no error)=w310) -> (queue out=w312:refnum<queue>, element=w304:refnum<class "BME_DG_System.lvclass">, error out=w306:errorcluster)  [unwired: 1 in, 1 out]
        n112 = call "Get Chnl by Name.vi"("BME_DG_System in"=w304, "Chnl Name"=w303, "error in (no error)"=w306) -> ("BME_DG_System out"=w307:refnum<class "BME_DG_System.lvclass">, "BME_DG_Chnl"=w301:refnum<class "BME_DG_Chnl.lvclass">, "Owner DG"=w300:refnum<class "BME_DG_Base.lvclass">, "error out"=w305:errorcluster)  [unwired: 7 in, 2 out]
        n113 = call-dynamic "Read objChnls.vi"("BME_DG_Base in"=w300) -> ("objChnls"=w299:refnum<class "BME_DG_Chnl.lvclass">[])  [unwired: 7 in, 3 out]
        n114 = for {
          tunnel: w299 -> [w318] mode=indexing
          tunnel: [w317] -> w298 mode=indexing
          n115 = call-dynamic "Read DelayFormula.vi"("BME_DG_Chnl in"=w318) -> ("DelayFormula"=w317:string)  [unwired: 8 in, 2 out]
        }
        n116 = call-dynamic "Read DelayFormula.vi"("BME_DG_Chnl in"=w301) -> ("DelayFormula"=w302:string)  [unwired: 8 in, 2 out]
        n117 = local write "DelayFormulas"(w298) -> ()
        n118 = local write "DelayFormula"(w302) -> ()
        n119 = Enqueue Element(queue=w312, element=w307, error in (no error)=w305) -> (queue out=w309:refnum<queue>, error out=w308:errorcluster)  [unwired: 1 in, 1 out]
      }
      event #7 {
        n120 = event-data() -> ()  [unwired: 1 in, 1 out]
        n121 = Dequeue Element(queue=w330, error in (no error)=w328) -> (queue out=w329:refnum<queue>, element=w323:refnum<class "BME_DG_System.lvclass">, error out=w327:errorcluster)  [unwired: 1 in, 1 out]
        n122 = call "ResetModuloCounters.vi"("error in (no error)"=w320, "Enum"=enum16{"Slaves only", "Slaves & Master"}."Slaves & Master", "BME_DG_System in"=w323) -> ("error out"=w321:errorcluster, "BME_DG_System out"=w322:refnum<class "BME_DG_System.lvclass">)  [unwired: 7 in]
        n123 = Enqueue Element(queue=w329, element=w322, error in (no error)=w327) -> (queue out=w325:refnum<queue>, error out=w326:errorcluster)  [unwired: 1 in, 1 out]
      }
      event #8 {
        n124 = event-data() -> ()  [unwired: 1 in, 1 out]
        n125 = property on="Selected Card" class="Ring (strict)"() -> ("Strings []"=w350:string[], "Value"=w349:u16)  [unwired: 2 in, 2 out]
        n126 = Dequeue Element(queue=w339, error in (no error)=w338) -> (queue out=w336:refnum<queue>, element=w337:refnum<class "BME_DG_System.lvclass">, error out=w335:errorcluster)  [unwired: 1 in, 1 out]
        n127 = Index Array(array=w350, index=w349) -> (element=w348:string)
        n128 = call "Get DG by LogicalName.vi"("error in (no error)"=w347, "LogicalName"=w348, "BME_DG_System in"=w337) -> ("error out"=w345:errorcluster, "found?"=w341:bool, "BME_DG_Base.lvclass"=w346:refnum<class "BME_DG_Base.lvclass">, "BME_DG_System out"=w342:refnum<class "BME_DG_System.lvclass">)  [unwired: 5 in]
        n129 = case shown="True" w341 {
          tunnel: w346 -> [w354 w361]
          tunnel: w345 -> [w353 w359]
          tunnel: [w353 w363] -> w344
          tunnel: [w354 w362] -> w343
          frame #0 {
            n130 = property on="Activate" class="Bool (strict)"("Value"=FALSE ("Activate"), "DisabledEnum"=T9."Disabled and Grayed Out" ("Disabled")) -> ()  [unwired: 2 in, 2 out]
          }
          frame #1 {
            n131 = call-dynamic "Read IsActive.vi"("error in (no error)"=w359, "BME_DG_Base in"=w361) -> ("error out"=w358:errorcluster, "Active?"=w357:bool, "BME_DG_Base out"=w360:refnum<class "BME_DG_Base.lvclass">)  [unwired: 7 in]
            n132 = Not(x=w357) -> (.not. x?=w355:bool)
            n133 = case shown="True" w357 {
              tunnel: [w367 w369] -> w363
              tunnel: [w366 w370] -> w362
              tunnel: w360 -> [w365 w371]
              tunnel: w358 -> [w364 w368]
              frame #0 {
                n134 = call-dynamic "Activate.vi"("error in (no error)"=w364, "BME_DG_Base in"=w365) -> ("error out"=w367:errorcluster, "BME_DG_Base out"=w366:refnum<class "BME_DG_Base.lvclass">)  [unwired: 8 in]
              }
              frame #1 {
                n135 = call-dynamic "Deactivate.vi"("error in (no error)"=w368, "BME_DG_Base in"=w371) -> ("error out"=w369:errorcluster, "BME_DG_Base out"=w370:refnum<class "BME_DG_Base.lvclass">)  [unwired: 8 in]
              }
            }
            n136 = property on="Activate" class="Bool (strict)"("Value"=w355, "DisabledEnum"=T9."Enabled" ("Disabled")) -> ()  [unwired: 2 in, 2 out]
          }
        }
        n137 = call "Write DG.vi"("error in (no error)"=w344, "BME_DG_Base"=w343, "BME_DG_System in"=w342) -> ("error out"=w340:errorcluster, "BME_DG_System out"=w334:refnum<class "BME_DG_System.lvclass">)  [unwired: 7 in]
        n138 = Enqueue Element(queue=w336, element=w334, error in (no error)=w335) -> (queue out=w333:refnum<queue>, error out=w332:errorcluster)  [unwired: 1 in, 1 out]
      }
      event #9 {
        n139 = event-data() -> ()  [unwired: 1 in, 1 out]
        n140 = property on="Selected Chnl" class="Ring (strict)"() -> ("Strings []"=w382:string[], "Value"=w383:u16)  [unwired: 2 in, 2 out]
        n141 = Index Array(array=w382, index=w383) -> (element=w379:string)
        n142 = local read "ChnParam2write"() -> (w378:T4)
        n143 = local read "TriggerModulo"() -> (w377:u32)
        n144 = Bundle By Name(cluster=w380, "ChnlName"=w379, "ChnParam2write"=w378, "TriggerModulo"=w377) -> (w375:T5)
        n145 = Enqueue Element(queue=w376, element=w375, error in (no error)=w374) -> (queue out=w373:refnum<queue>, error out=w372:errorcluster)  [unwired: 1 in, 1 out]
      }
    }
    "error out" <- w167
  }
  n146 = while {
    tunnel: w67 -> [w393]
    shift-right: [w391] -> w90
    shift-left: w66 -> [w392]
    shift-right: [w388] -> w74
    shift-left: w60 -> [w390]
    tunnel: w77 -> [w387]
    tunnel: w76 -> [w386]
    stop <- w395 stop-if-true
    n147 = case shown="True" "ReadStatus" {
      tunnel: w393 -> [_ w424]
      tunnel: w392 -> [w398 w423]
      tunnel: [w398 w422] -> w391
      tunnel: w390 -> [w397 w420]
      tunnel: [w397 w406] -> w388
      tunnel: w387 -> [_ w410]
      tunnel: w386 -> [_ w409]
      frame #0 {
        n148 = Wait Until Next ms Multiple(millisecond multiple=u32 200) -> ()  [unwired: 1 out]
      }
      frame #1 {
        n149 = Dequeue Element(queue=w424, error in (no error)=w423) -> (queue out=w425:refnum<queue>, element=w421:refnum<class "BME_DG_System.lvclass">, error out=w426:errorcluster)  [unwired: 1 in, 1 out]
        n150 = Wait Until Next ms Multiple(millisecond multiple=u32 10) -> ()  [unwired: 1 out]
        n151 = call "ReadHWState.vi"("error in (no error)"=w420, "BME_DG_System in"=w421) -> ("error out"=w419:errorcluster, "Interrupts"=w415:u32[], "BME_DG_System out"=w418:refnum<class "BME_DG_System.lvclass">)  [unwired: 7 in]
        n152 = Or(x=u32 8192, y=w415) -> (x .or. y?=→"Interrupts":u32[])
        n153 = call "Read TriggersTillShot.vi"("error in (no error)"=w419, "BME_DG_System in"=w418) -> ("error out"=w411:errorcluster, "TriggerCounters"=→"TriggerCounters":i32[], "RemainingTriggers"=w417:T6, "BME_DG_System out"=w412:refnum<class "BME_DG_System.lvclass">)  [unwired: 6 in]
        n154 = call "CountsTillNextCommonTrigger.vi"("error in (no error)"=w411, "BME_DG_System in"=w412) -> ("error out"=w408:errorcluster, "LeastCommonMult"=w403:i32, "CountsRemains"=w404:i32, "BME_DG_System out"=w407:refnum<class "BME_DG_System.lvclass">)  [unwired: 6 in]
        "CountsRemains" <- w404
        n155 = Transpose 2D Array(2D array=w417) -> (transposed array=→"RemainingTriggers":T6)
        n156 = Equal?(x=w404, y=w403) -> (x = y?=w402:bool)
        n157 = case shown="No Error" w408 {
          selector: w408 -> [w430 w443]
          tunnel: w410 -> [w433 _]
          tunnel: w409 -> [w432 _]
          tunnel: w407 -> [w431 w444]
          tunnel: [w429 w443] -> w406
          tunnel: [w428 w444] -> w405
          tunnel: w402 -> [w427 _]
          frame #0 {
            n158 = case shown="True" w427 {
              tunnel: w433 -> [_ w442]
              tunnel: w432 -> [_ w441]
              tunnel: w431 -> [w435 w440]
              tunnel: w430 -> [w434 w438]
              tunnel: [w434 w437] -> w429
              tunnel: [w435 w436] -> w428
              frame #0 {
              }
              frame #1 {
                n159 = Flush Queue(queue=w442, error in (no error)=w441) -> (remaining elements=w439:T10)  [unwired: 2 out]
                n160 = call "Update Chnls.vi"("error in (no error)"=w438, "ChnlSettings"=w439, "BME_DG_System in"=w440) -> ("error out"=w437:errorcluster, "BME_DG_System out"=w436:refnum<class "BME_DG_System.lvclass">)  [unwired: 7 in]
              }
            }
          }
          frame #1 {
          }
        }
        n161 = Enqueue Element(queue=w425, element=w405, error in (no error)=w426) -> (error out=w422:errorcluster)  [unwired: 1 in, 2 out]
      }
    }
    n162 = Unbundle By Name(w388) -> ("status"=w394:bool)
    n163 = Or(x=w394, y="stop 2") -> (x .or. y?=w395:bool)
  }
  n164 = while {
    tunnel: w67 -> [w449]
    shift-right: [w446] -> w64
    shift-left: w66 -> [w448]
    stop <- w451 stop-if-true
    n165 = case shown="True" "Aknowledge interrupts" {
      tunnel: w449 -> [_ w461]
      tunnel: w448 -> [w453 w460]
      tunnel: [w453 w459] -> w446
      frame #0 {
      }
      frame #1 {
        n166 = Dequeue Element(queue=w461, error in (no error)=w460) -> (queue out=w458:refnum<queue>, element=w457:refnum<class "BME_DG_System.lvclass">, error out=w456:errorcluster)  [unwired: 1 in, 1 out]
        n167 = call "AcknowledgeInterrupts.vi"("error in (no error)"=w456, "BME_DG_System in"=w457) -> ("error out"=w454:errorcluster, "BME_DG_System out"=w455:refnum<class "BME_DG_System.lvclass">)  [unwired: 8 in]
        n168 = Enqueue Element(queue=w458, element=w455, error in (no error)=w454) -> (error out=w459:errorcluster)  [unwired: 1 in, 2 out]
      }
    }
    n169 = Wait Until Next ms Multiple(millisecond multiple=u32 500) -> ()  [unwired: 1 out]
    n170 = Unbundle By Name(w446) -> ("status"=w450:bool)
    n171 = Or(x=w450, y="stop 3") -> (x .or. y?=w451:bool)
  }
  n172 = call <vilib>:"Merge Errors.vi"("error in 3 (no error)"=w64, "error in 2 (no error)"=w90, "error in 1 (no error)"=w91) -> ("error out"=w92:errorcluster)  [unwired: 4 in]
  n173 = call <vilib>:"Merge Errors.vi"("error in 2 (no error)"=w74, "error in 1 (no error)"=w75) -> ("error out"=w73:errorcluster)  [unwired: 5 in]
  n174 = Release Queue(queue=w79, force destroy? (F)=TRUE, error in (no error)=w73) -> (error out=w48:errorcluster)  [unwired: 2 out]
  n175 = Release Queue(queue=w93, error in (no error)=w92) -> (error out=w49:errorcluster)  [unwired: 1 in, 2 out]
  n176 = call <vilib>:"Merge Errors.vi"("error in 2 (no error)"=w48, "error in 1 (no error)"=w49) -> ("error out"=→"stop error":errorcluster)  [unwired: 5 in]
